vi "RTD Settings.vi"(8 "error in (no error)":errorcluster, 11 "TT Configuration In":T1={"physical channels"="cDAQ2Mod4/ai0", "name to assign"="Temp1", "units"=10143} {"units" items=["Deg C"=10143, "Deg F"=10144, "Kelvins"=10325, "Deg R"=10145, "From Custom Scale"=10065]}) -> (0 "error out":errorcluster, 3 "TT Configuration Out":T1={"physical channels"="cDAQ2Mod4/ai0", "name to assign"="Temp1", "units"=10143} {"units" items=["Deg C"=10143, "Deg F"=10144, "Kelvins"=10325, "Deg R"=10145, "From Custom Scale"=10065]})   [LabVIEW 2021, in "RTD.lvlib"]
uses:
  RTD.lvlib
panel:
  in  "Cancel":bool
  in  "OK Button":bool
  in  "TT Configuration":T1={"physical channels"="cDAQ2Mod4/ai0", "name to assign"="Temp1", "units"=10143} {"units" items=["Deg C"=10143, "Deg F"=10144, "Kelvins"=10325, "Deg R"=10145, "From Custom Scale"=10065]}
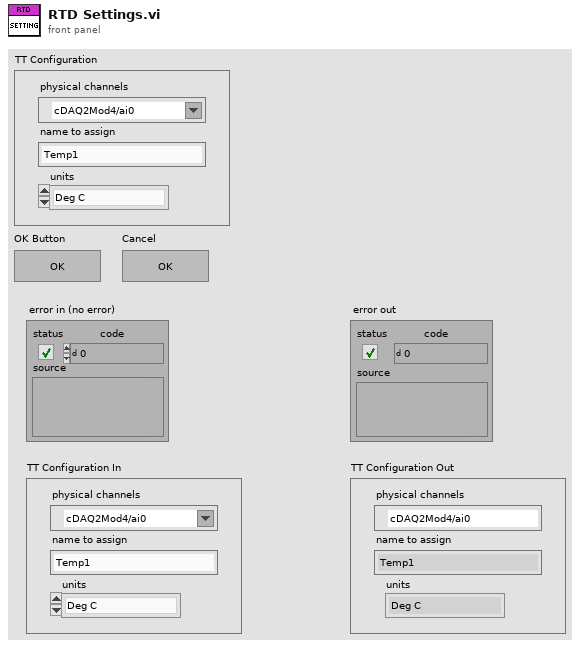
[diagram p1: front panel]
types:
  T1 = cluster{"physical channels":tag, "name to assign":string, "units":i32}
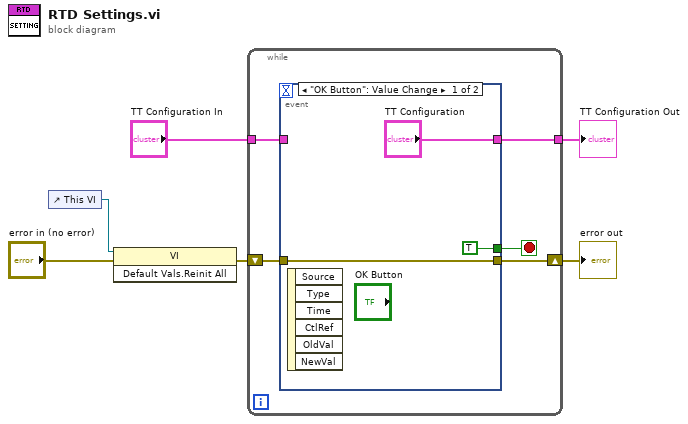
[diagram p0: block diagram]
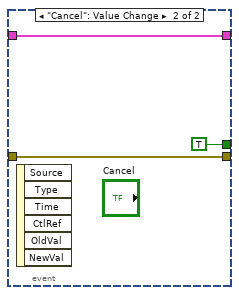
[diagram p2: hidden frame]
diagram:
  n1 = control-ref of="This VI"() -> (w3:refnum<vi>)
  n2 = invoke class="VI" method="Default Vals.Reinit All"(reference=w3, error in="error in (no error)") -> (error out=w1:errorcluster)  [unwired: 1 in, 2 out]
  n3 = while {
    tunnel: [w11] -> w6
    shift-right: [w10] -> w5
    shift-left: w1 -> [w9]
    tunnel: "TT Configuration In" -> [w7]
    stop <- w8 stop-if-true
    n4 = event shown="[0] \"OK Button\": Value Change" {
      selector: _ -> [_ _]
      dyn-events: _ -> [_ _]
      timeout: _ -> [_ _]
      tunnel: ["TT Configuration" w15] -> w11
      tunnel: [w14 w17] -> w10
      tunnel: w9 -> [w14 w17]
      tunnel: [TRUE TRUE] -> w8
      tunnel: w7 -> [_ w15]
      event "OK Button": Value Change {
        n5 = event-data() -> ()  [unwired: 1 in, 6 out]
      }
      event "Cancel": Value Change {
        n6 = event-data() -> ()  [unwired: 1 in, 6 out]
      }
    }
  }
  "TT Configuration Out" <- w6
  "error out" <- w5
